vi "EncodeUInt64.vi"(1 "Data In":u64[](array[numeric])) -> (0 "Data Out":u8[](array[numeric]))   [LabVIEW 2014, in "navX Library v1 (deprecated).lvlib"]
uses:
  navX Library v1 (deprecated).lvlib
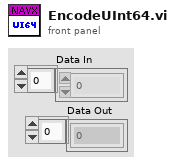
[diagram p1: front panel]
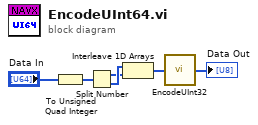
[diagram p0: block diagram]
diagram:
  n1 = To Unsigned Quad Integer(1:"Data In") -> (0:w1:u64[])
  n2 = Split Number(x=w1) -> (hi(x)=w4:u32[], lo(x)=w5:u32[])
  n3 = Interleave 1D Arrays(w5, w4) -> (w3:u32[])
  n4 = call "EncodeUInt32.vi"("Data In"=w3) -> ("Data Out"=→"Data Out":u8[])
